vi "G Object to Standard PLC Byte Stream.vi"(6 "Byte Length":i32, 8 "error in (no error)":errorcluster, 9 "PLC Type":T1, 10 "Value":variant, 11 "TwinCAT ADS in":refnum<class "TwinCAT ADS.lvclass">) -> (0 "error out":errorcluster, 2 "Byte Stream":u8[](array[numeric]), 3 "TwinCAT ADS out":refnum<class "TwinCAT ADS.lvclass">)   [LabVIEW 2018, in "TwinCAT ADS.lvclass"]
uses:
  TwinCAT ADS.lvclass
  Controls/PLC Type.ctl
  TwinCAT.Ads
  ebfc1059-5ad7-41af-9a32-6ba056cec1e2.vi
  6e01a951-886b-41b5-8cd1-fdd71fd1a533.vi
  09c7a0ef-3209-4624-b801-f77696e71225.vi
  d245b078-1949-470f-93ac-23e830eec426.vi
  0fd4fbf3-4a18-432c-8f70-6a5c8fef8454.vi
  afdb5a5e-237c-4be5-828e-15f510cf6cea.vi
  185a6e12-4d7d-4ad7-9936-0525adb2f85e.vi
  88229fb8-b58c-494b-bd2b-fea6e0d0ed1b.vi
  e57df404-389c-41d0-a67c-37c75754ab31.vi
  d0ee652c-9b86-46ed-9065-57d03aa8de3e.vi
  886bf0b9-f01c-4a44-b2e2-abccc7b97bfa.vi
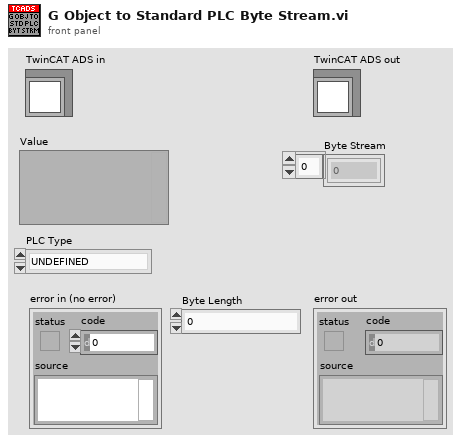
[diagram p1: front panel]
types:
  T1 = typedef "TwinCAT ADS.lvclass/PLC Type.ctl" = enum16{"UNDEFINED", "INT", "DINT", "REAL", "LREAL", "SINT", "BYTE", "UINT", "UDINT", "LINT", "ULINT", "STRING", "WSTRING", "BOOL", "TIME", "LTIME", "DATE", "DT", "TOD", "ARRAY", "STRUCT", "JAGGED ARRAY", "USER DEFINED"}
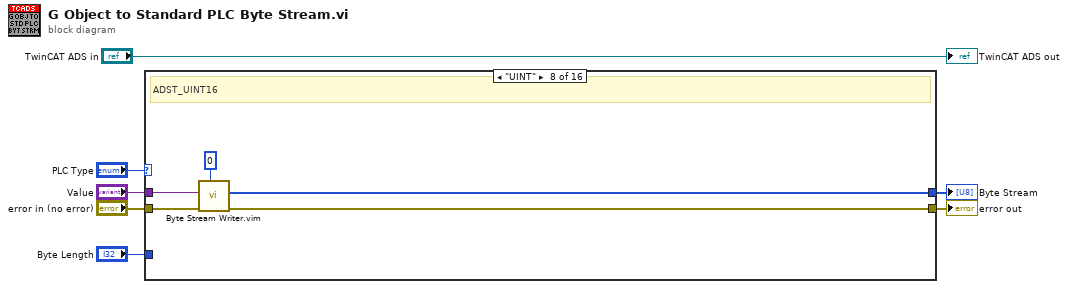
[diagram p0: block diagram]
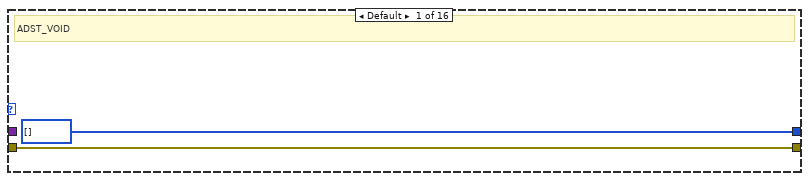
[diagram p2: hidden frame]
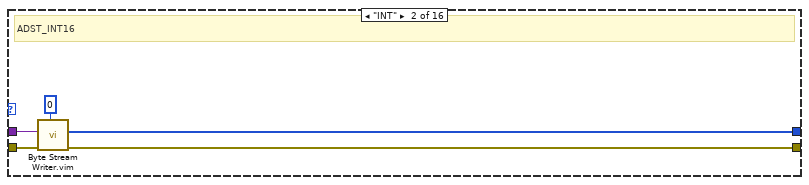
[diagram p3: hidden frame]
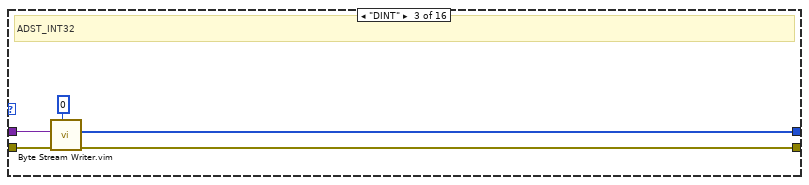
[diagram p4: hidden frame]
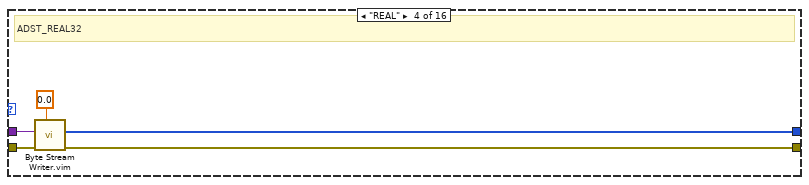
[diagram p5: hidden frame]
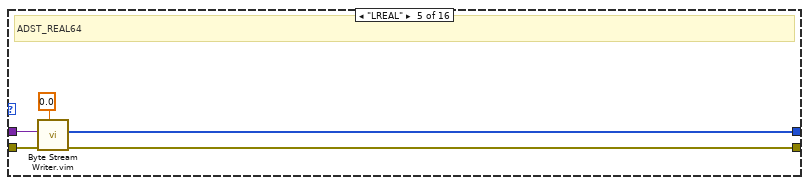
[diagram p6: hidden frame]
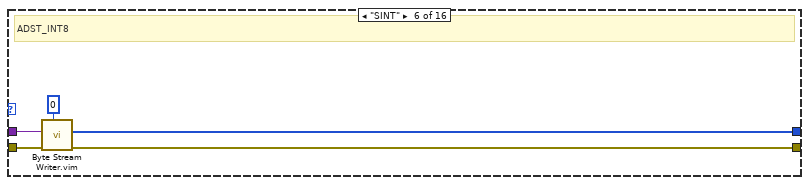
[diagram p7: hidden frame]
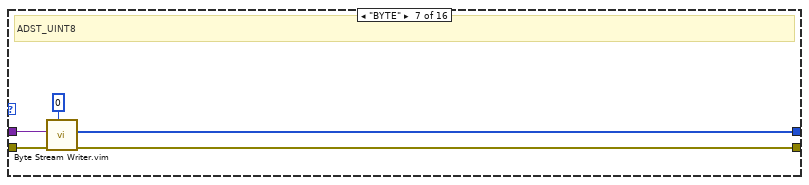
[diagram p8: hidden frame]
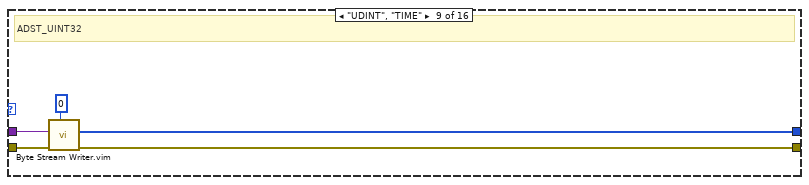
[diagram p9: hidden frame]
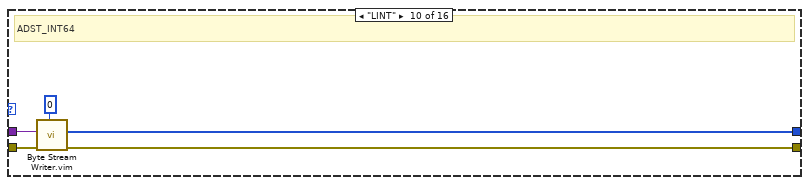
[diagram p10: hidden frame]
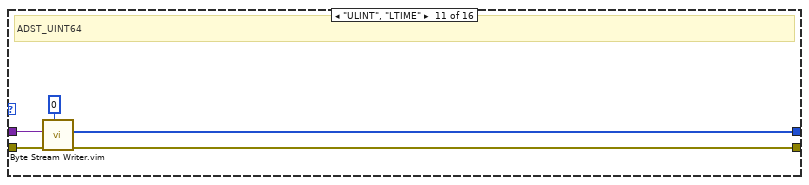
[diagram p11: hidden frame]
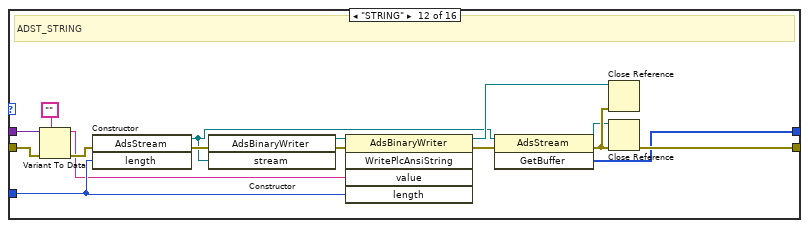
[diagram p12: hidden frame]
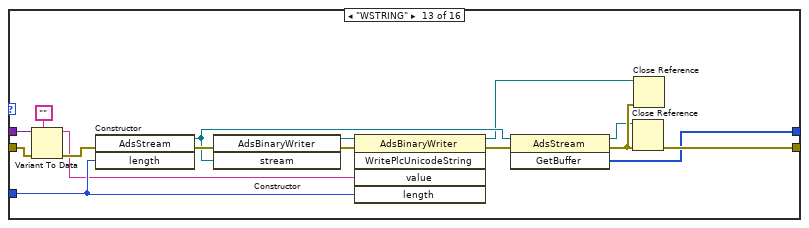
[diagram p13: hidden frame]
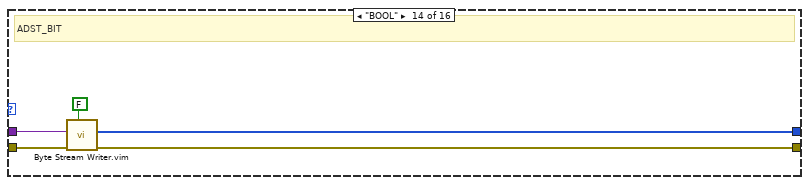
[diagram p14: hidden frame]
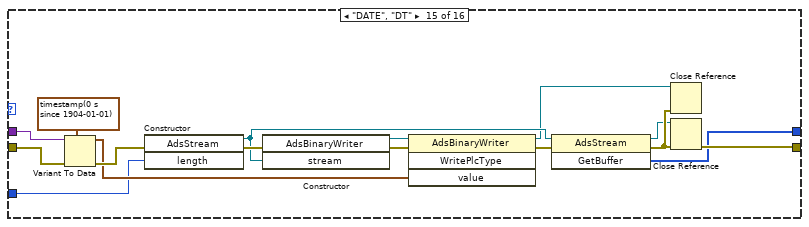
[diagram p15: hidden frame]
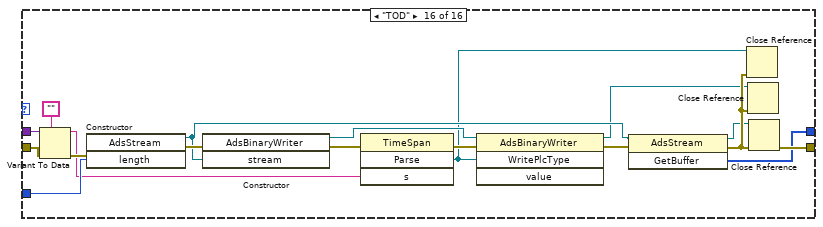
[diagram p16: hidden frame]
diagram:
  n1 = case shown="\"UINT\"" "PLC Type" {
    tunnel: "error in (no error)" -> [w9 w14 w19 w24 w29 w34 w39 w44 w49 w54 w59 w71 w79 w96 w108 w120]
    tunnel: [w9 w11 w17 w21 w26 w31 w36 w41 w48 w51 w56 w75 w83 w93 w109 w115] -> w6
    tunnel: "Value" -> [_ w13 w18 w23 w28 w33 w38 w43 w45 w53 w58 w69 w78 w95 w107 w118]
    tunnel: [u8[] [] ("Byte Stream") w10 w15 w20 w25 w30 w35 w40 w47 w50 w55 w61 w82 w92 w98 w114] -> w4
    tunnel: "Byte Length" -> [_ _ _ _ _ _ _ _ _ _ _ w67 w81 _ w97 w116]
    frame Default {
      # "ADST_VOID"
    }
    frame "INT" {
      # "ADST_INT16"
      n2 = call "Byte Stream Writer.vim"("Type"=i16 0, "error in (no error)"=w14, "Value"=w13) -> ("error out"=w11:errorcluster, "Byte Stream"=w10:u8[])  [unwired: 7 in]
    }
    frame "DINT" {
      # "ADST_INT32"
      n3 = call "Byte Stream Writer.vim"("Type"=0, "error in (no error)"=w19, "Value"=w18) -> ("error out"=w17:errorcluster, "Byte Stream"=w15:u8[])  [unwired: 7 in]
    }
    frame "REAL" {
      # "ADST_REAL32"
      n4 = call "Byte Stream Writer.vim"("Type"=sgl 0.0, "error in (no error)"=w24, "Value"=w23) -> ("error out"=w21:errorcluster, "Byte Stream"=w20:u8[])  [unwired: 7 in]
    }
    frame "LREAL" {
      # "ADST_REAL64"
      n5 = call "Byte Stream Writer.vim"("Type"=0.0, "error in (no error)"=w29, "Value"=w28) -> ("error out"=w26:errorcluster, "Byte Stream"=w25:u8[])  [unwired: 7 in]
    }
    frame "SINT" {
      # "ADST_INT8"
      n6 = call "Byte Stream Writer.vim"("Type"=i8 0, "error in (no error)"=w34, "Value"=w33) -> ("error out"=w31:errorcluster, "Byte Stream"=w30:u8[])  [unwired: 7 in]
    }
    frame "BYTE" {
      # "ADST_UINT8"
      n7 = call "Byte Stream Writer.vim"("Type"=u8 0, "error in (no error)"=w39, "Value"=w38) -> ("error out"=w36:errorcluster, "Byte Stream"=w35:u8[])  [unwired: 7 in]
    }
    frame "UINT" {
      # "ADST_UINT16"
      n8 = call "Byte Stream Writer.vim"("Type"=u16 0, "error in (no error)"=w44, "Value"=w43) -> ("error out"=w41:errorcluster, "Byte Stream"=w40:u8[])  [unwired: 7 in]
    }
    frame "UDINT", "TIME" {
      # "ADST_UINT32"
      n9 = call "Byte Stream Writer.vim"("Type"=u32 0, "error in (no error)"=w49, "Value"=w45) -> ("error out"=w48:errorcluster, "Byte Stream"=w47:u8[])  [unwired: 7 in]
    }
    frame "LINT" {
      # "ADST_INT64"
      n10 = call "Byte Stream Writer.vim"("Type"=i64 0, "error in (no error)"=w54, "Value"=w53) -> ("error out"=w51:errorcluster, "Byte Stream"=w50:u8[])  [unwired: 7 in]
    }
    frame "ULINT", "LTIME" {
      # "ADST_UINT64"
      n11 = call "Byte Stream Writer.vim"("Type"=u64 0, "error in (no error)"=w59, "Value"=w58) -> ("error out"=w56:errorcluster, "Byte Stream"=w55:u8[])  [unwired: 7 in]
    }
    frame "STRING" {
      # "ADST_STRING"
      n12 = Variant To Data(error in=w71, type="", Variant=w69) -> (data=w66:string, error out=w70:errorcluster)
      n13 = constructor class="AdsStream"(error in=w70, "length"=w67) -> (reference out=w60:refnum<k24>, error out=w74:errorcluster)  [unwired: 2 in, 2 out]
      n14 = constructor class="AdsBinaryWriter"(error in=w74, "stream"=w60) -> (reference out=w72:refnum<k24>, error out=w73:errorcluster)  [unwired: 2 in, 2 out]
      n15 = invoke class="AdsBinaryWriter" method="WritePlcAnsiString"(reference=w72, error in=w73, "value"=w66, "length"=w67) -> (reference out=w62:refnum<k24>, error out=w65:errorcluster)  [unwired: 1 in, 3 out]
      n16 = invoke class="AdsStream" method="GetBuffer"(reference=w60, error in=w65) -> (reference out=w63:refnum<k24>, error out=w64:errorcluster, "GetBuffer"=w61:u8[])  [unwired: 1 in]
      n17 = Close Reference(reference=w62, error in (no error)=w64) -> ()  [unwired: 1 out]
      n18 = Close Reference(reference=w63, error in (no error)=w64) -> (error out=w75:errorcluster)
    }
    frame "WSTRING" {
      n19 = Variant To Data(error in=w79, type="", Variant=w78) -> (data=w76:string, error out=w77:errorcluster)
      n20 = constructor class="AdsStream"(error in=w77, "length"=w81) -> (reference out=w87:refnum<k24>, error out=w89:errorcluster)  [unwired: 2 in, 2 out]
      n21 = constructor class="AdsBinaryWriter"(error in=w89, "stream"=w87) -> (reference out=w91:refnum<k24>, error out=w90:errorcluster)  [unwired: 2 in, 2 out]
      n22 = invoke class="AdsBinaryWriter" method="WritePlcUnicodeString"(reference=w91, error in=w90, "value"=w76, "length"=w81) -> (reference out=w84:refnum<k24>, error out=w88:errorcluster)  [unwired: 1 in, 3 out]
      n23 = invoke class="AdsStream" method="GetBuffer"(reference=w87, error in=w88) -> (reference out=w85:refnum<k24>, error out=w86:errorcluster, "GetBuffer"=w82:u8[])  [unwired: 1 in]
      n24 = Close Reference(reference=w85, error in (no error)=w86) -> (error out=w83:errorcluster)
      n25 = Close Reference(reference=w84, error in (no error)=w86) -> ()  [unwired: 1 out]
    }
    frame "BOOL" {
      # "ADST_BIT"
      n26 = call "Byte Stream Writer.vim"("Type"=FALSE, "error in (no error)"=w96, "Value"=w95) -> ("error out"=w93:errorcluster, "Byte Stream"=w92:u8[])  [unwired: 7 in]
    }
    frame "DATE", "DT" {
      n27 = Variant To Data(error in=w108, type=timestamp(0 s since 1904-01-01), Variant=w107) -> (data=w104:timestamp, error out=w105:errorcluster)
      n28 = constructor class="AdsStream"(error in=w105, "length"=w97) -> (reference out=w102:refnum<k24>, error out=w110:errorcluster)  [unwired: 2 in, 2 out]
      n29 = constructor class="AdsBinaryWriter"(error in=w110, "stream"=w102) -> (reference out=w112:refnum<k24>, error out=w111:errorcluster)  [unwired: 2 in, 2 out]
      n30 = invoke class="AdsBinaryWriter" method="WritePlcType"(reference=w112, error in=w111, "value"=w104) -> (reference out=w99:refnum<k24>, error out=w103:errorcluster)  [unwired: 1 in, 2 out]
      n31 = invoke class="AdsStream" method="GetBuffer"(reference=w102, error in=w103) -> (reference out=w100:refnum<k24>, error out=w101:errorcluster, "GetBuffer"=w98:u8[])  [unwired: 1 in]
      n32 = Close Reference(reference=w99, error in (no error)=w101) -> ()  [unwired: 1 out]
      n33 = Close Reference(reference=w100, error in (no error)=w101) -> (error out=w109:errorcluster)
    }
    frame "TOD" {
      n34 = Variant To Data(error in=w120, type="", Variant=w118) -> (data=w113:string, error out=w119:errorcluster)
      n35 = constructor class="AdsStream"(error in=w119, "length"=w116) -> (reference out=w125:refnum<k24>, error out=w130:errorcluster)  [unwired: 2 in, 2 out]
      n36 = constructor class="AdsBinaryWriter"(error in=w130, "stream"=w125) -> (reference out=w127:refnum<k24>, error out=w128:errorcluster)  [unwired: 2 in, 2 out]
      n37 = invoke class="TimeSpan" method="Parse"(error in=w128, "s"=w113) -> (error out=w129:errorcluster, "Parse"=w121:refnum<k24>)  [unwired: 2 in, 2 out]
      n38 = invoke class="AdsBinaryWriter" method="WritePlcType"(reference=w127, error in=w129, "value"=w121) -> (reference out=w122:refnum<k24>, error out=w126:errorcluster)  [unwired: 1 in, 2 out]
      n39 = invoke class="AdsStream" method="GetBuffer"(reference=w125, error in=w126) -> (reference out=w123:refnum<k24>, error out=w124:errorcluster, "GetBuffer"=w114:u8[])  [unwired: 1 in]
      n40 = Close Reference(reference=w121, error in (no error)=w124) -> ()  [unwired: 1 out]
      n41 = Close Reference(reference=w122, error in (no error)=w124) -> ()  [unwired: 1 out]
      n42 = Close Reference(reference=w123, error in (no error)=w124) -> (error out=w115:errorcluster)
    }
  }
  "error out" <- w6
  "Byte Stream" <- w4
  "TwinCAT ADS out" <- "TwinCAT ADS in"
